vi "editConfiguration.vi"(8 "error in (no error)":errorcluster, 11 "ConfigurationTestParameters in":refnum<class "ConfigurationTestParameters.lvclass">) -> (0 "error out":errorcluster, 2 "cancelIsTrue out":bool, 3 "ConfigurationTestParameters out":refnum<class "ConfigurationTestParameters.lvclass">)   [LabVIEW 2016, in "ConfigurationTestParameters.lvclass"]
uses:
  ConfigurationTestParameters.lvclass
  ConfigurationTestParameters.lvclass/ConfigurationTestParameters.ctl
  displayConfigurableElements.vi
  Common_ConfigurationEditor/ConfigurationEditor.lvclass
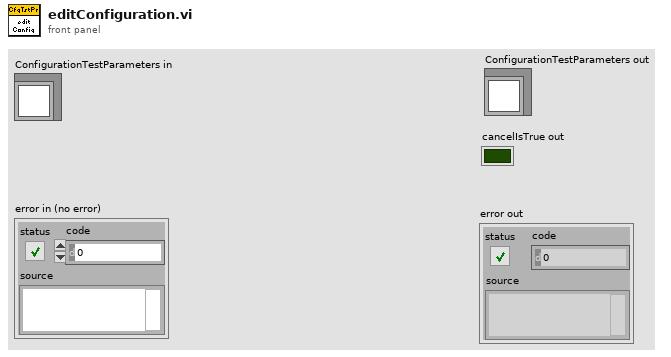
[diagram p1: front panel]
types:
  T1 = enum32{"Bad", "Idle", "Run top level", "Running"}
  T2 = enum32{"Invalid", "Standard", "Closed", "Hidden", "Minimized", "Maximized"}
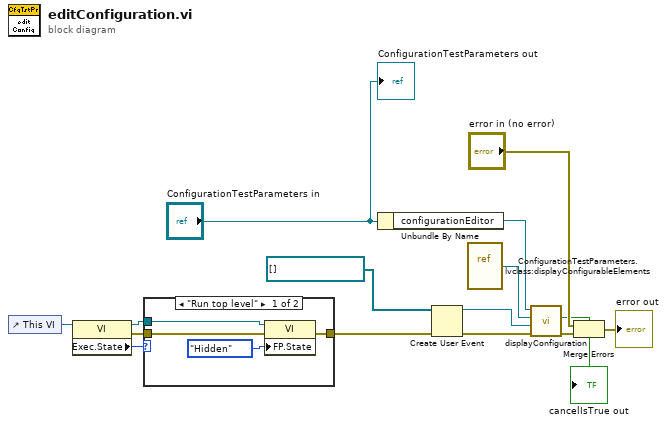
[diagram p0: block diagram]
diagram:
  n1 = control-ref of="This VI"() -> (w11:refnum<vi>)
  n2 = property class="VI"(reference=w11) -> (reference out=w9:refnum<vi>, error out=w7:errorcluster, "Exec.State"=w10:T1)  [unwired: 1 in]
  n3 = case shown="\"Run top level\"" w10 {
    tunnel: w9 -> [w18 _]
    tunnel: [w17 w20] -> w8
    tunnel: w7 -> [w16 w20]
    frame "Run top level" {
      n4 = property class="VI"(reference=w18, error in=w16, "FP.State"=T2."Hidden" ("Front Panel Window:State")) -> (error out=w17:errorcluster)  [unwired: 1 out]
    }
    frame "Running", Default {
    }
  }
  n5 = Unbundle By Name("ConfigurationTestParameters in") -> ("configurationEditor"=w3:refnum<class "ConfigurationEditor.lvclass">)
  n6 = Create User Event(user event datatype=refnum<vi>[] [] ("cfgCtrlRefs"), error in=w8) -> (user event=w13:refnum<user-event>, error out=w12:errorcluster)
  n7 = vi-ref "ConfigurationTestParameters.lvclass:displayConfigurableElements.vi"() -> (w15:refnum<vi>)
  n8 = call "displayConfiguration.vi"("error in (no error)"=w12, "ctrlRefArrayUsrEvnt"=w13, "configurableElementsVI"=w15, "ConfigurationEditor in"=w3) -> ("error out"=w5:errorcluster, "cancelIsTrue out"=→"cancelIsTrue out":bool)  [unwired: 5 in, 1 out]
  n9 = Merge Errors("error in (no error)", w5) -> (→"error out":errorcluster)
  "ConfigurationTestParameters out" <- "ConfigurationTestParameters in"
